vi "Get Notifier Ref.vi"(8 "error in (no error)":errorcluster, 11 "iCVT_Item in":refnum<class "iCVT_Item.lvclass">) -> (0 "error out":errorcluster, 3 "iCVT_Item out":refnum<class "iCVT_Item.lvclass">)   [LabVIEW 2024]
uses:
  iCVT_Item.lvclass
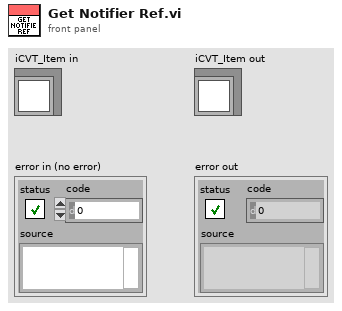
[diagram p1: front panel]
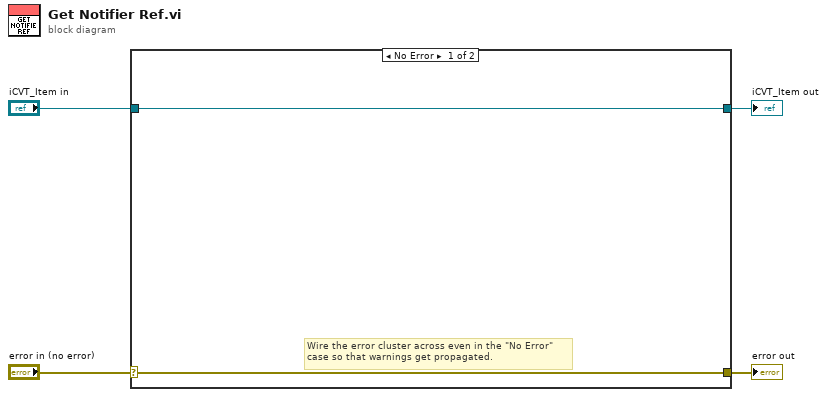
[diagram p0: block diagram]
diagram:
  n1 = case shown="No Error" "error in (no error)" {
    selector: "error in (no error)" -> [w5 w8]
    tunnel: [w5 w8] -> w3
    tunnel: [w6 w7] -> w1
    tunnel: "iCVT_Item in" -> [w6 w7]
    frame No Error {
      # "Wire the error cluster across even in the \"No Error\"\ncase so that warnings get propagated."
    }
    frame Error {
    }
  }
  "error out" <- w3
  "iCVT_Item out" <- w1
